vi "Find Channel by SN - SimpleStat.vi"(6 "Search Channel":string, 7 "Model Number":string, 8 "error in (no error)":errorcluster, 9 "Statistics Data":T1, 10 "Query Parameters":T3, 11 "Serial Number":T4) -> (0 "error out":errorcluster, 1 "Statistics Data out":T1)   [LabVIEW 2011]
uses:
  TDMS/TDMS Serial Number.ctl
  TDMS/TDMS File.ctl
  TDMS/TDMS Run.ctl
  TDMS/TDMS Channel (Sxx).ctl
  database/Fields/Field Record.ctl
  database/Fields/Field DataTypes.ctl
  database/Fields/Field NextItem.ctl
  Datasheet Analysis Parameters.ctl
  Statistics Data.ctl
  CGI SimpleStat Results.ctl
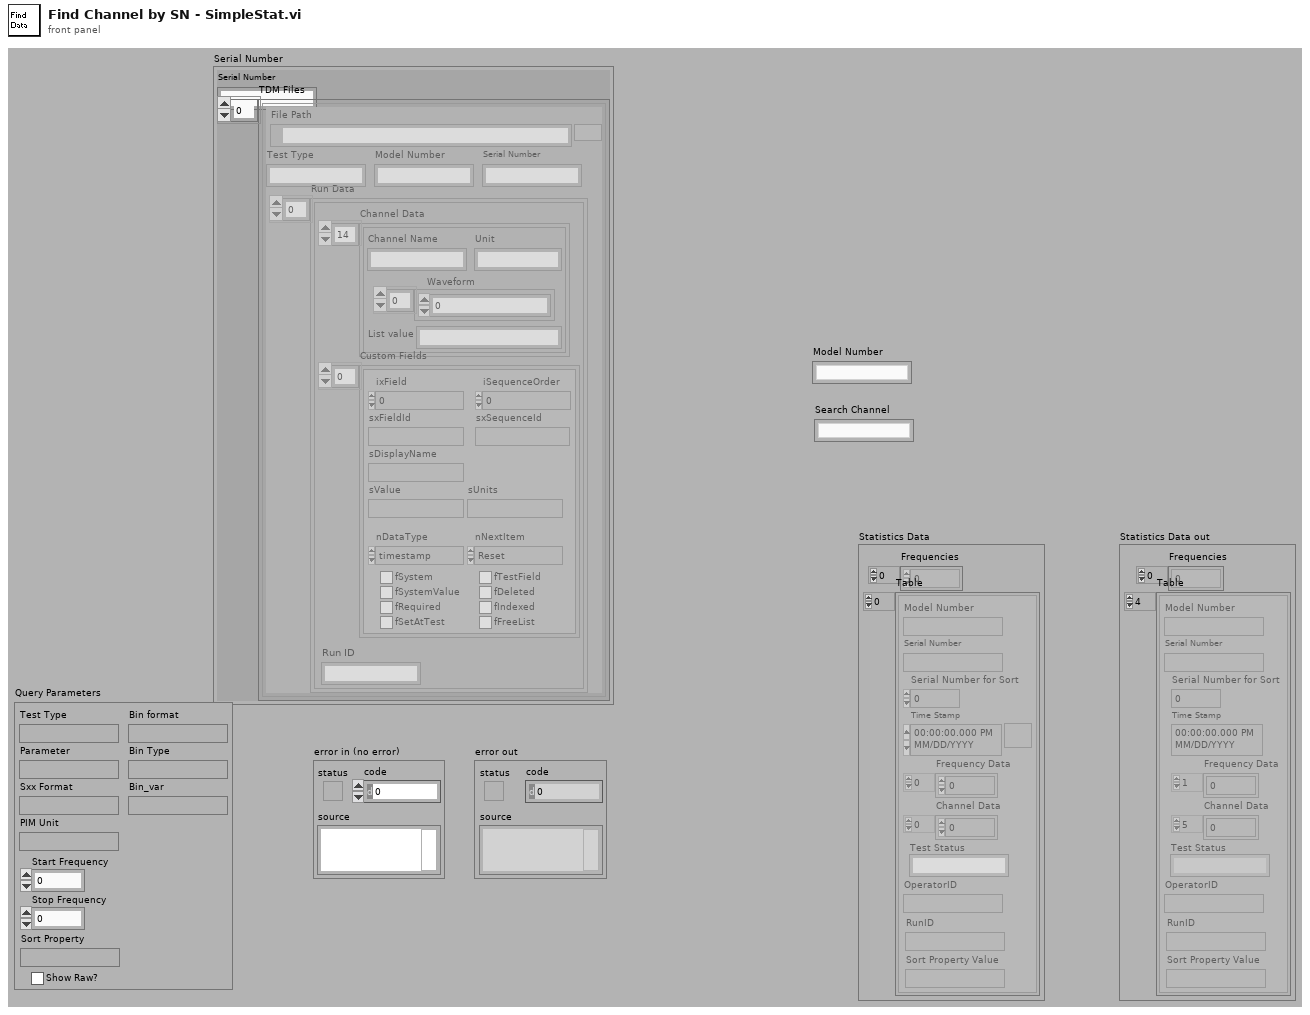
[diagram p1: front panel]
types:
  T1 = typedef "Statistics Data.ctl" = cluster{"Table":T2[], "Frequencies":dbl[]}
  T2 = typedef "CGI SimpleStat Results.ctl" = cluster{"Model Number":string, "Serial Number for Sort":i32, "Serial Number":string, "Time Stamp":timestamp, "Channel Data":dbl[], "Test Status":string, "OperatorID":string, "Frequency Data":dbl[], "RunID":string, "Sort Property Value":string}
  T3 = typedef "Datasheet Analysis Parameters.ctl" = cluster{"Test Type":string, "Parameter":string, "Sxx Format":string, "PIM Unit":string, "Start Frequency":dbl, "Stop Frequency":dbl, "Sort Property":string, "Show Raw?":bool, "Bin format":string, "Bin Type":string, "Bin_var":string}
  T4 = typedef "TDMS Serial Number.ctl" = cluster{"Serial Number":string, "TDM Files":T5[]}
  T5 = typedef "TDMS File.ctl" = cluster{"File Path":path, "Run Data":T6[], "Serial Number":string, "Model Number":string, "Test Type":string}
  T6 = typedef "TDMS Run.ctl" = cluster{"Channel Data":T7[], "Custom Fields":T8[], "Run ID":string}
  T7 = typedef "TDMS Channel (Sxx).ctl" = cluster{"Channel Name":string, "Waveform":dbl[], "Unit":string, "List value":string}
  T8 = typedef "Field Record.ctl" = cluster{"ixField":i32, "iSequenceOrder":i32, "sxFieldId":string, "sxSequenceId":string, "sDisplayName":string, "sValue":string, "sUnits":string, "nDataType":T9, "nNextItem":T10, "fSystem":bool, "fSystemValue":bool, "fRequired":bool, "fSetAtTest":bool, "fTestField":bool, "fDeleted":bool, "fIndexed":bool, "fFreeList":bool}
  T9 = typedef "Field DataTypes.ctl" = enum32{"text", "numeric", "list", "timestamp", "boolean"}
  T10 = typedef "Field NextItem.ctl" = enum32{"Reset", "Retain", "Auto-Increment"}
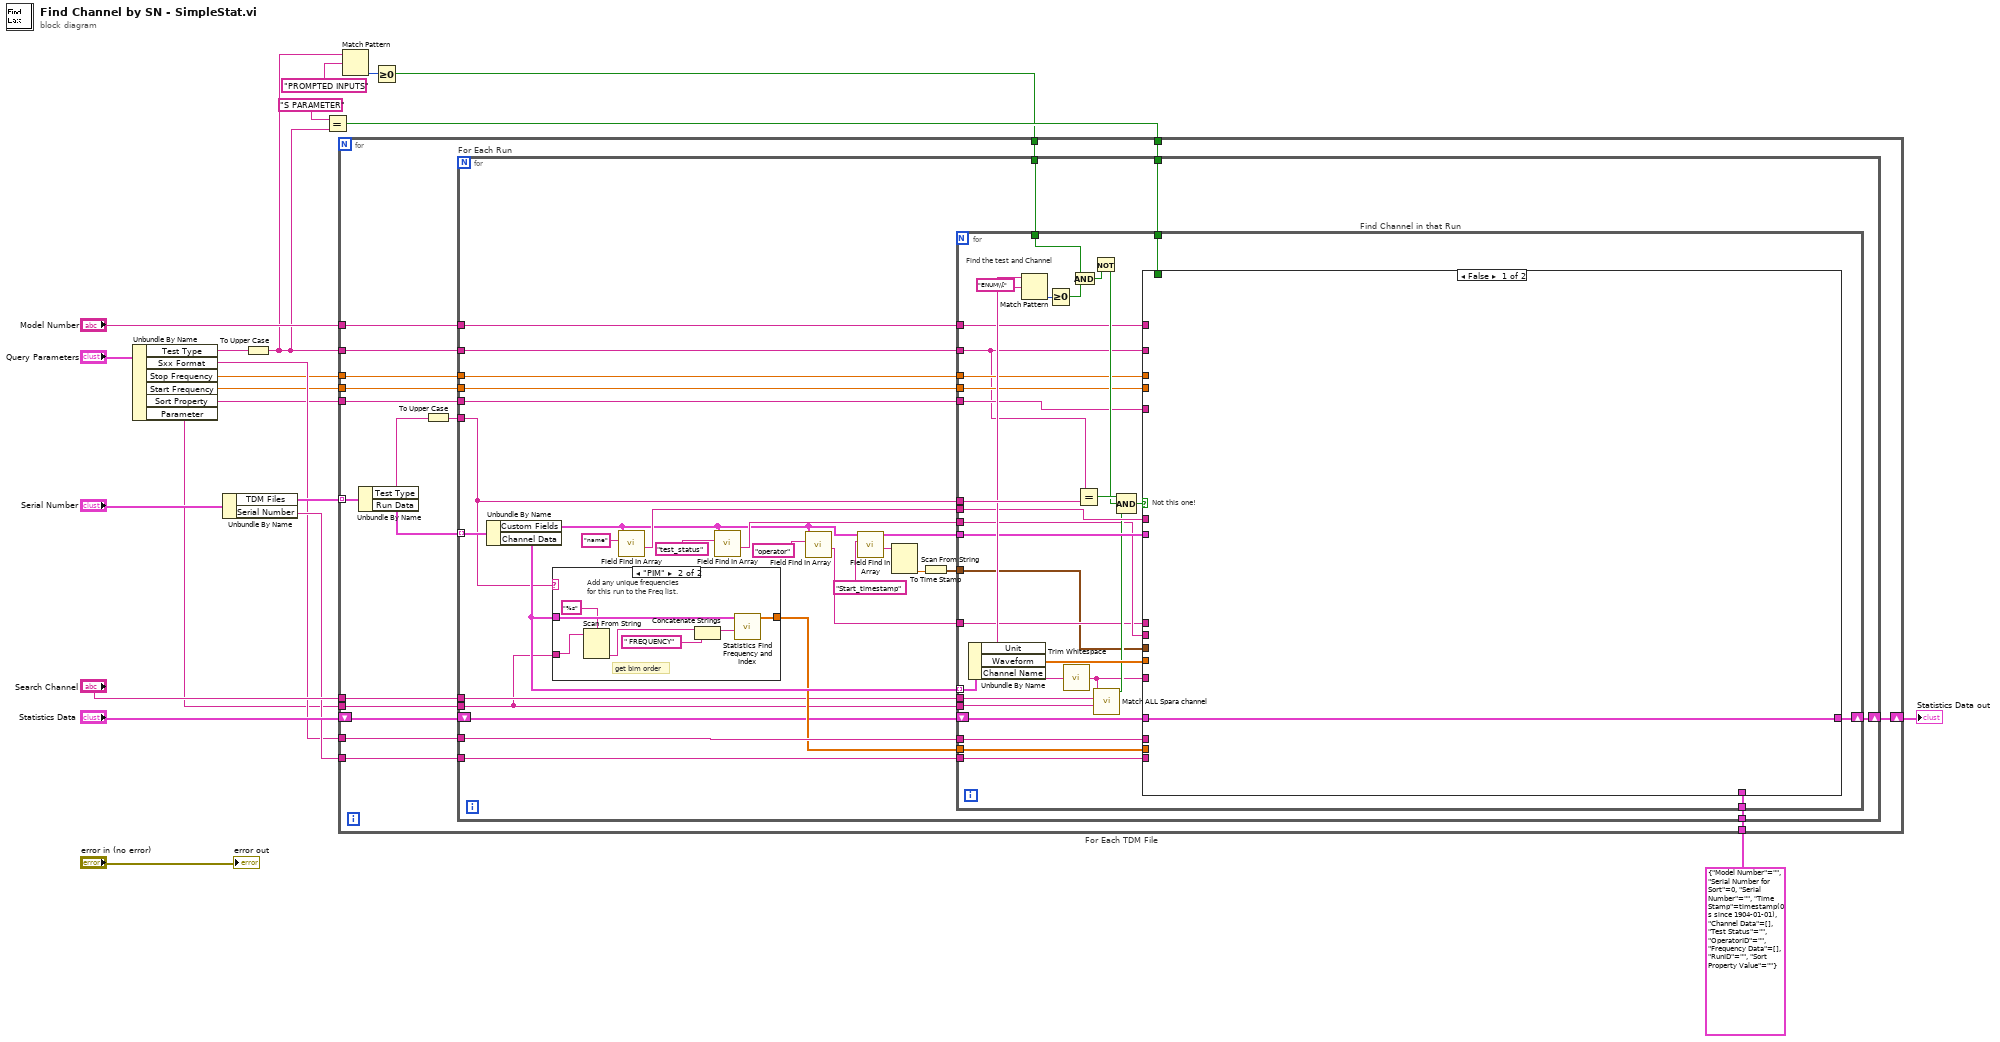
[diagram p0: block diagram]
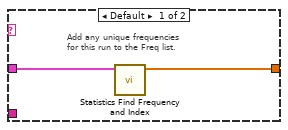
[diagram p2: hidden frame]
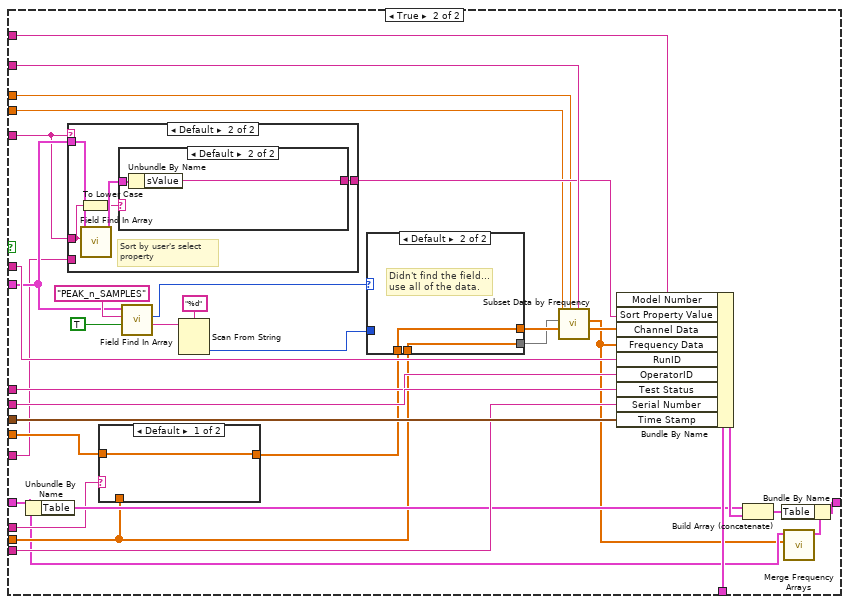
[diagram p3: hidden frame]
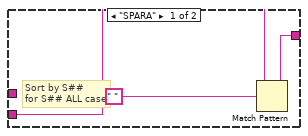
[diagram p4: hidden frame]
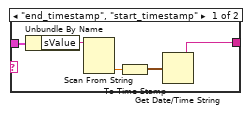
[diagram p5: hidden frame]
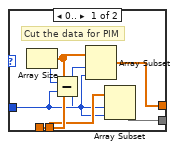
[diagram p6: hidden frame]
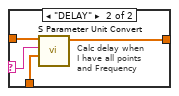
[diagram p7: hidden frame]
diagram:
  n1 = Unbundle By Name("Query Parameters") -> ("Test Type"=w6:string, "Sxx Format"=w12:string, "Stop Frequency"=w9:dbl, "Start Frequency"=w8:dbl, "Sort Property"=w7:string, "Parameter"=w1:string)
  n2 = Unbundle By Name("Serial Number") -> ("TDM Files"=w20:T5[], "Serial Number"=w13:string)
  n3 = To Upper Case(1:w6) -> (0:w2:string)
  n4 = Equal?(x="S PARAMETER", y=w2) -> (x = y?=w14:bool)
  n5 = Match Pattern(string=w2, regular expression="PROMPTED INPUTS" ("x")) -> (offset past match=w4:i32)  [unwired: 4 out]
  n6 = Greater Or Equal To 0?(x=w4) -> (x >= 0?=w3:bool)
  n7 = for "For Each TDM File" {
    shift-right: [w39] -> w18
    shift-left: "Statistics Data" -> [w38]
    tunnel: w20 -> [w37] mode=indexing
    tunnel: "Search Channel" -> [w36]
    tunnel: T2 {"Model Number"="", "Serial Number for Sort"=0, "Serial Number"="", "Time Stamp"=timestamp(0 s since 1904-01-01), "Channel Data"=[], "Test Status"="", "OperatorID"="", "Frequency Data"=[], "RunID"="", "Sort Property Value"=""} ("Sample Results") -> [w34]
    tunnel: w14 -> [w33]
    tunnel: w13 -> [w32]
    tunnel: w12 -> [w31]
    tunnel: w3 -> [w30]
    tunnel: "Model Number" -> [w29]
    tunnel: w2 -> [w28]
    tunnel: w9 -> [w27]
    tunnel: w8 -> [w26]
    tunnel: w7 -> [w25]
    tunnel: w1 -> [w24]
    n8 = Unbundle By Name(w37) -> ("Test Type"=w35:string, "Run Data"=w40:T6[])
    n9 = To Upper Case(1:w35) -> (0:w23:string)
    n10 = for "For Each Run" {
      tunnel: w40 -> [w69] mode=indexing
      shift-right: [w68] -> w39
      shift-left: w38 -> [w53]
      tunnel: w36 -> [w58]
      tunnel: w23 -> [w59]
      tunnel: w34 -> [w67]
      tunnel: w33 -> [w66]
      tunnel: w32 -> [w65]
      tunnel: w31 -> [w64]
      tunnel: w30 -> [w63]
      tunnel: w29 -> [w60]
      tunnel: w28 -> [w57]
      tunnel: w27 -> [w56]
      tunnel: w26 -> [w55]
      tunnel: w25 -> [w54]
      tunnel: w24 -> [w41]
      n11 = Unbundle By Name(w69) -> ("Custom Fields"=w46:T8[], "Channel Data"=w62:T7[])
      n12 = case shown="\"PIM\"" w59 {
        tunnel: w62 -> [w71 w78]
        tunnel: [w70 w76] -> w61
        tunnel: w41 -> [_ w74]
        frame Default {
          # "Add any unique frequencies\nfor this run to the Freq list."
          n13 = call "Statistics Find Frequency and Index.vi"("Channel Data"=w71) -> ("Frequency Array"=w70:dbl[])  [unwired: 1 in, 9 out]
        }
        frame "PIM" {
          # "get bim order"
          # "Add any unique frequencies\nfor this run to the Freq list."
          n14 = Scan From String(format string="%s", input string=w74) -> (output 1=w72:string)  [unwired: 2 in, 4 out]
          n15 = Concatenate Strings(w72, " FREQUENCY" ("FieldID or Display Name(\"\")")) -> (w77:string)
          n16 = call "Statistics Find Frequency and Index.vi"("Frequency Channel Name"=w77, "Channel Data"=w78) -> ("Frequency Array"=w76:dbl[])  [unwired: 1 in, 8 out]
        }
      }
      n17 = call "Field Find In Array.vi"("FieldID or Display Name(\"\")"="name" ("FieldID or Display Name(\"\")"), "Field Array"=w46) -> ("sValue"=w51:string)  [unwired: 1 in, 8 out]
      n18 = call "Field Find In Array.vi"("FieldID or Display Name(\"\")"="test_status" ("FieldID or Display Name(\"\")"), "Field Array"=w46) -> ("sValue"=w49:string)  [unwired: 1 in, 8 out]
      n19 = call "Field Find In Array.vi"("FieldID or Display Name(\"\")"="operator" ("FieldID or Display Name(\"\")"), "Field Array"=w46) -> ("sValue"=w45:string)  [unwired: 1 in, 8 out]
      n20 = call "Field Find In Array.vi"("FieldID or Display Name(\"\")"="Start_timestamp" ("FieldID or Display Name(\"\")"), "Field Array"=w46) -> ("sValue"=w44:string)  [unwired: 1 in, 8 out]
      n21 = Scan From String(input string=w44) -> (output 1=w43:dbl)  [unwired: 3 in, 4 out]
      n22 = To Time Stamp(1:w43) -> (0:w42:timestamp)
      n23 = for "Find Channel in that Run" {
        tunnel: w62 -> [w91] mode=indexing
        shift-right: [w112] -> w68
        shift-left: w53 -> [w90]
        tunnel: w58 -> [w86]
        tunnel: w59 -> [w107]
        tunnel: w67 -> [w106]
        tunnel: w66 -> [w105]
        tunnel: w65 -> [w104]
        tunnel: w64 -> [w87]
        tunnel: w63 -> [w99]
        tunnel: w61 -> [w96]
        tunnel: w60 -> [w95]
        tunnel: w51 -> [w94]
        tunnel: w46 -> [w93]
        tunnel: w57 -> [w79]
        tunnel: w56 -> [w81]
        tunnel: w55 -> [w80]
        tunnel: w54 -> [w92]
        tunnel: w41 -> [w85]
        tunnel: w49 -> [w84]
        tunnel: w45 -> [w83]
        tunnel: w42 -> [w82]
        # "Find the test and Channel"
        n24 = Unbundle By Name(w91) -> ("Unit"=w102:string, "Waveform"=w111:dbl[], "Channel Name"=w110:string)
        n25 = Match Pattern(string=w102, regular expression="ENUM\\[") -> (offset past match=w101:i32)  [unwired: 4 out]
        n26 = Greater Or Equal To 0?(x=w101) -> (x >= 0?=w100:bool)
        n27 = call <vilib>:"Trim Whitespace.vi"("string"=w110) -> ("trimmed string"=w88:string)  [unwired: 1 in]
        n28 = And(x=w99, y=w100) -> (x .and. y?=w98:bool)
        n29 = Equal?(x=w79, y=w107) -> (x = y?=w108:bool)
        n30 = Not(x=w98) -> (.not. x?=w97:bool)
        n31 = call "Match ALL Spara channel.vi"("Spara Type Channel"=w85, "Search Channel"=w86, "Channel Name"=w88) -> ("Load This?"=w89:bool)  [unwired: 8 out]
        n32 = Compound Arithmetic op=AND(w108, w97, w89) -> (w109:bool)
        n33 = case shown="False" w109 {
          tunnel: w90 -> [w113 w123]
          tunnel: [w113 w142] -> w112
          tunnel: w111 -> [_ w137]
          tunnel: w82 -> [_ w147]
          tunnel: w106 -> [_ w144]
          tunnel: w105 -> [_ _]
          tunnel: w104 -> [_ w143]
          tunnel: w87 -> [_ w138]
          tunnel: w84 -> [_ w140]
          tunnel: w83 -> [_ w139]
          tunnel: w96 -> [_ w132]
          tunnel: w95 -> [_ w115]
          tunnel: w94 -> [_ w136]
          tunnel: w93 -> [_ w126]
          tunnel: w79 -> [_ w127]
          tunnel: w92 -> [_ w119]
          tunnel: w88 -> [_ w120]
          tunnel: w81 -> [_ w117]
          tunnel: w80 -> [_ w116]
          frame False {
            # "Not this one!"
          }
          frame True {
            n34 = Unbundle By Name(w123) -> ("Table"=w141:T2[])
            n35 = case shown="Default" w119 {
              tunnel: w126 -> [_ w155]
              tunnel: w119 -> [_ w152]
              tunnel: [w148 w153] -> w125
              tunnel: w120 -> [w149 _]
              frame "SPARA" {
                # "Sort by S##\nfor S## ALL case"
                n36 = Match Pattern(string=w149, regular expression=" ") -> (before substring=w148:string)  [unwired: 4 out]
              }
              frame Default {
                # "Sort by user's select\nproperty"
                n37 = To Lower Case(string=w152) -> (all lower case string=w151:string)
                n38 = call "Field Find In Array.vi"("FieldID or Display Name(\"\")"=w152, "Field Array"=w155) -> ("Field"=w154:T8)  [unwired: 1 in, 8 out]
                n39 = case shown="Default" w151 {
                  tunnel: w154 -> [w160 w162]
                  tunnel: [w156 w161] -> w153
                  frame "end_timestamp", "start_timestamp" {
                    n40 = Unbundle By Name(w160) -> ("sValue"=w159:string)
                    n41 = Scan From String(input string=w159) -> (output 1=w158:dbl)  [unwired: 3 in, 4 out]
                    n42 = To Time Stamp(1:w158) -> (0:w157:timestamp)
                    n43 = Get Date/Time String(seconds (now)=w157) -> (date string=w156:string)  [unwired: 3 out]
                  }
                  frame Default {
                    n44 = Unbundle By Name(w162) -> ("sValue"=w161:string)
                  }
                }
              }
            }
            n45 = case shown="Default" w138 {
              selector: w138 -> [_ w173]
              tunnel: w137 -> [w172 w176]
              tunnel: [w172 w175] -> w134
              tunnel: w132 -> [_ w174]
              frame Default {
              }
              frame "DELAY" {
                # "Calc delay when\nI have all points\nand Frequency"
                n46 = call "S Parameter Unit Convert.vi"("Frequency Array"=w174, "Format"=w173, "Waveform IN"=w176) -> ("Waveform out"=w175:dbl[])  [unwired: 8 out]
              }
            }
            n47 = call "Field Find In Array.vi"("by DisplayName? (f, by FieldId)"=TRUE, "FieldID or Display Name(\"\")"="PEAK_n_SAMPLES" ("Field_ID (\"\")"), "Field Array"=w126) -> ("sValue"=w114:string, "Index"=w133:i32)  [unwired: 7 out]
            n48 = Scan From String(format string="%d", input string=w114) -> (output 1=w130:i32)  [unwired: 2 in, 4 out]
            n49 = case shown="Default" w133 {
              tunnel: w134 -> [w167 w171]
              tunnel: [w168 w171] -> w129
              tunnel: w132 -> [w166 w170]
              tunnel: [w165 w170] -> w124
              tunnel: w130 -> [w164 _]
              frame 0.. {
                # "Cut the data for PIM"
                n50 = Array Size(array=w167) -> (size(s)=w169:i32)
                n51 = Subtract(x=w169, y=w164) -> (x-y=w163:i32)
                n52 = Array Subset(array=w167, index=w163, length=w164) -> (w168:dbl[])
                n53 = Array Subset(array=w166, index=w163, length=w164) -> (w165:dbl[])
              }
              frame Default {
                # "Didn't find the field...\nuse all of the data."
              }
            }
            n54 = call "Subset Data by Frequency.vi"("Test Type"=w127, "Stop Frequency"=w117, "Channel Data"=w129, "Frequency Data"=w124, "Start Frequency"=w116) -> ("Channel Data 2"=w128:dbl[], "Frequency Data 2"=w121:dbl[])  [unwired: 5 out]
            n55 = Bundle By Name(cluster=w144, "Model Number"=w115, "Sort Property Value"=w125, "Channel Data"=w128, "Frequency Data"=w121, "RunID"=w136, "OperatorID"=w139, "Test Status"=w140, "Serial Number"=w143, "Time Stamp"=w147) -> (w146:T2)
            n56 = Build Array (concatenate)(w141, w146) -> (w145:T2[])
            n57 = call "Merge Frequency Arrays.vi"("New Frequencies to merge"=w121, "Statistics Data"=w123) -> ("Statistics Data 2"=w122:T1)  [unwired: 9 out]
            n58 = Bundle By Name(cluster=w122, "Table"=w145) -> (w142:T1)
          }
        }
      }
    }
  }
  "Statistics Data out" <- w18
  "error out" <- "error in (no error)"
